vi "Get All Folder VI Data.vi"(8 "error in (no error)":errorcluster, 11 "Folder Path":path) -> (0 "error out":errorcluster, 3 "VI Data":T1[](array[typedef]))   [LabVIEW 2020, in "VI Properties Editor.lvlib"]
doc: "Gets all VI data from a folder located at <B>Path</B>."
uses:
  VI Properties Editor.lvlib
  CTLs/Control Properties.ctl
  <vilib>/picture/picture.llb/imagedata.ctl
  CTLs/VI Properties.ctl
  CTLs/VI Data.ctl
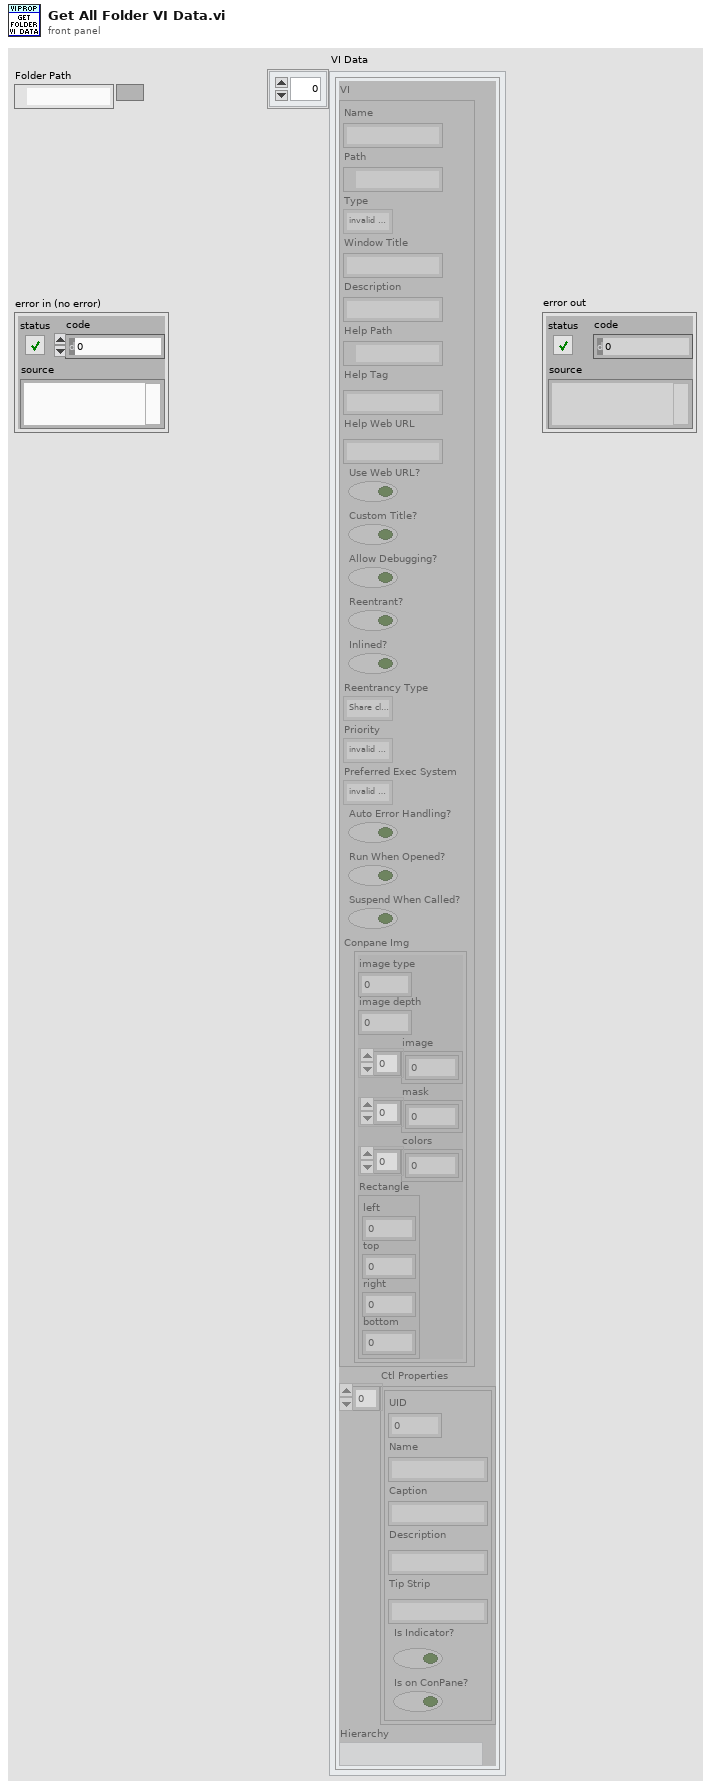
[diagram p1: front panel]
types:
  T1 = typedef "VI Properties Editor.lvlib/VI Data.ctl" = cluster{"VI":T2, "Ctl Properties":T4[], "Hierarchy":string}
  T2 = typedef "VI Properties Editor.lvlib/VI Properties.ctl" = cluster{"Name":string, "Path":path, "Type":enum32{"invalid VI type", "Standard VI", "Control VI", "Global VI", "Polymorphic VI", "Configuration VI", "SubSystem", "Facade VI", "Method VI", "Statechart Diagram VI"}, "Window Title":string, "Description":string, "Help Path":path, "Help Tag":string, "Help Web URL":string, "Use Web URL?":bool, "Custom Title?":bool, "Allow Debugging?":bool, "Reentrant?":bool, "Inlined?":bool, "Reentrancy Type":enum16{"Share clones between instances", "Preallocate clone for each instance"}, "Priority":enum32{"invalid priority", "background priority", "normal priority", "above normal priority", "high priority", "time critical priority", "subroutine"}, "Preferred Exec System":enum32{"invalid execution system", "user interface", "standard", "instrument i/o", "data acquisition", "other 1", "other 2", "same as caller"}, "Auto Error Handling?":bool, "Run When Opened?":bool, "Suspend When Called?":bool, "Conpane Img":T3}
  T3 = typedef "imagedata.ctl" = cluster{"image type":i32, "image depth":i32, "image":u8[], "mask":u8[], "colors":u32[], "Rectangle":cluster{"left":i16, "top":i16, "right":i16, "bottom":i16}}
  T4 = typedef "VI Properties Editor.lvlib/Control Properties.ctl" = cluster{"UID":i32, "Name":string, "Caption":string, "Description":string, "Tip Strip":string, "Is Indicator?":bool, "Is on ConPane?":bool}
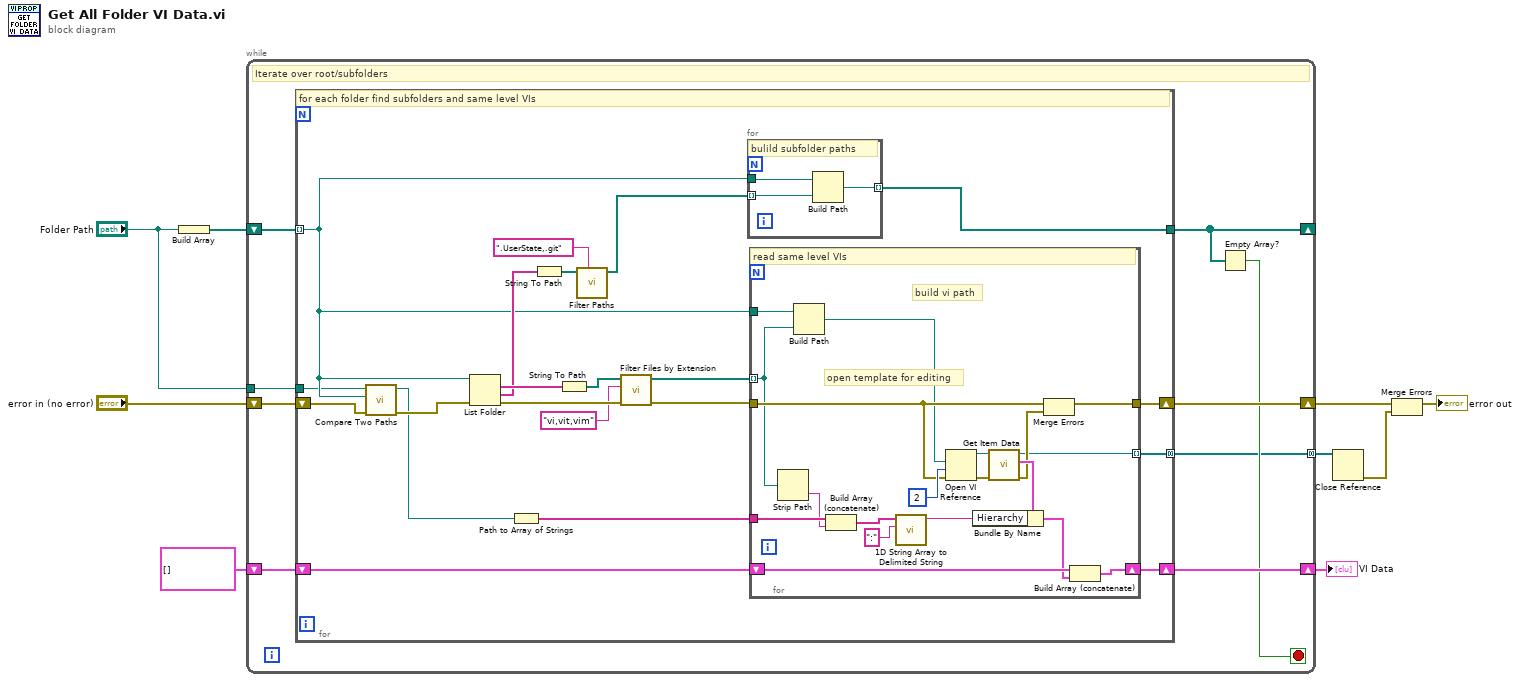
[diagram p0: block diagram]
diagram:
  n1 = Build Array("Folder Path") -> (w8:path[])
  n2 = while {
    shift-right: [w18] -> w3
    shift-left: "error in (no error)" -> [w15]
    shift-right: [w17] -> w5
    shift-left: T1[] [] ("VI Data") -> [w16]
    shift-right: [w13] -> _
    shift-left: w8 -> [w14]
    tunnel: "Folder Path" -> [w11]
    tunnel: [w10] -> w4 mode=concatenating
    stop <- w12 stop-if-true
    # "Iterate over root/subfolders"
    n3 = for {
      tunnel: w14 -> [w23] mode=indexing
      shift-right: [w34] -> w18
      shift-left: w15 -> [w25]
      shift-right: [w39] -> w17
      shift-left: w16 -> [w38]
      tunnel: [w35] -> w13
      tunnel: w11 -> [w22]
      tunnel: [w19] -> w10 mode=concatenating
      # "for each folder find subfolders and same level VIs"
      n4 = call <vilib>:"Compare Two Paths.vi"("error in (no error)"=w25, "Path 2"=w23, "Path 1"=w22) -> ("error out"=w24:errorcluster, "Relative Path from 1 to 2"=w21:path)  [unwired: 5 in, 2 out]
      n5 = List Folder(path=w23, error in=w24) -> (filenames=w37:string[], folder names=w29:string[], error out=w32:errorcluster)  [unwired: 2 in, 1 out]
      n6 = Path to Array of Strings(0:w21) -> (2:w20:string[])  [unwired: 1 out]
      n7 = String To Path(string=w29) -> (path=w27:path[])
      n8 = String To Path(string=w37) -> (path=w36:path[])
      n9 = call "Filter Paths.vi"("Argument"=".UserState,.git", "Paths"=w27) -> ("Filtered Path"=w28:path[])  [unwired: 9 in]
      n10 = call "Filter Files by Extension.vi"("error in (no error)"=w32, "Extensions"="vi,vit,vim", "Files"=w36) -> ("error out"=w31:errorcluster, "Files out"=w33:path[])  [unwired: 7 in]
      n11 = for {
        tunnel: w23 -> [w60]
        tunnel: w28 -> [w61] mode=indexing
        tunnel: [w59] -> w35 mode=indexing
        # "bulild subfolder paths"
        n12 = Build Path(base path=w60, name or relative path=w61) -> (appended path=w59:path)
      }
      n13 = for {
        tunnel: w31 -> [w54]
        tunnel: [w53] -> w34
        shift-right: [w55] -> w39
        shift-left: w38 -> [w51]
        tunnel: w33 -> [w44] mode=indexing
        tunnel: w23 -> [w52]
        tunnel: w20 -> [w47]
        tunnel: [w40] -> w19 mode=indexing
        # "build vi path"
        # "open template for editing"
        # "read same level VIs"
        n14 = Strip Path(path=w44) -> (name=w42:string)  [unwired: 1 out]
        n15 = Build Path(base path=w52, name or relative path=w44) -> (appended path=w49:path)
        n16 = Build Array (concatenate)(w47, w42) -> (w43:string[])
        n17 = call <vilib>:"1D String Array to Delimited String.vi"("delimiter"=":", "string array"=w43) -> ("delimited string"=w45:string)  [unwired: 9 in]
        n18 = Open VI Reference(vi path=w49, options=2, error in (no error)=w54) -> (vi reference=w56:refnum<vi>, error out=w57:errorcluster)  [unwired: 3 in]
        n19 = call "Get Item Data.vi"("error in (no error)"=w57, "VI Ref"=w56) -> ("error out"=w41:errorcluster, "VI Data"=w48:T1, "VI Ref out"=w40:refnum<vi>)  [unwired: 7 in]
        n20 = Bundle By Name(cluster=w48, "Hierarchy"=w45) -> (w50:T1)
        n21 = Merge Errors(w54, w41) -> (w53:errorcluster)
        n22 = Build Array (concatenate)(w51, w50) -> (w55:T1[])
      }
    }
    n23 = Empty Array?(array=w13) -> (empty?=w12:bool)
  }
  "VI Data" <- w5
  n24 = Close Reference(reference=w4) -> (error out=w2:errorcluster)  [unwired: 1 in]
  n25 = Merge Errors(w3, w2) -> (→"error out":errorcluster)
